vi "ex3_producer_consumer_deltat.vi"() -> ()   [LabVIEW 2022 SP3]
uses:
  C:/Program Files (x86)/National Instruments/LabVIEW 2022/examples/Connectivity/Python/support/PythonVersionsEnum.ctl
  pylabview/pythonq.lvlib
panel:
  out "delta_t_wv":dbl(graph)
  out "delta_t":dbl
  out "cur ref 2":string
  out "error out 2":errorcluster
  out "Wv 2":dbl(graph)
  out "cur ref":string
  out "count 1":i32
  in  "wait":u32=500
  out "Wv":dbl(graph)
  in  "stop":bool
  out "count 2":i32
  out "error out":errorcluster
  # "This example shows 2 connections to the python data ques, 1 to produce data, and one to consumer it, all in parrallel\n\nCreated by Jeff Morgan\nhttps://awakeniot.com/"
  # "https://github.com/jmor2000/labview_python_bridge"
  # "DATA IN"
  # "DATA OUT"
  # "DELTA T"
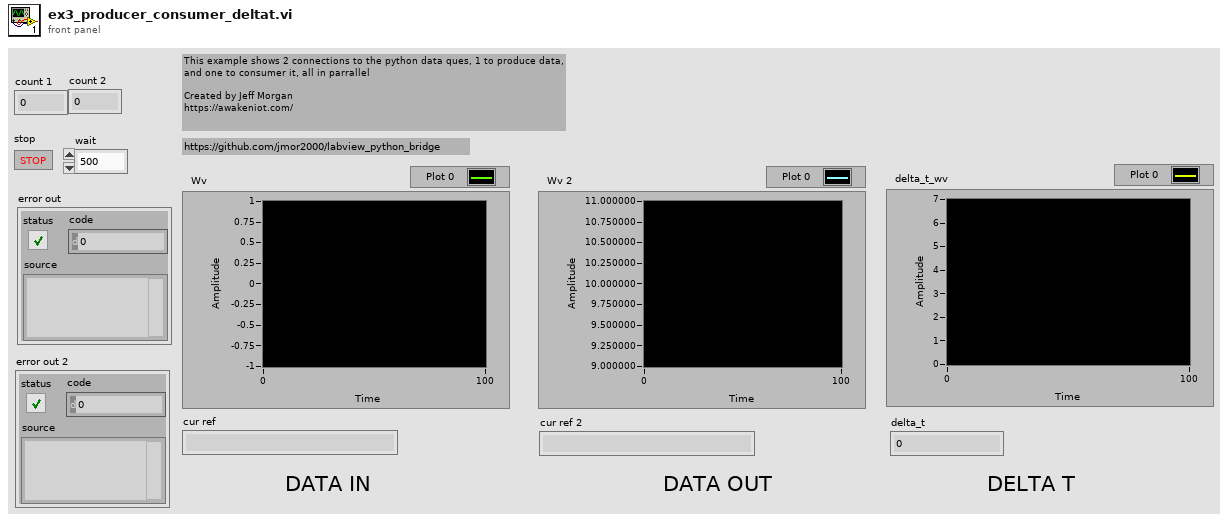
[diagram p1: front panel]
types:
  T1 = typedef "PythonVersionsEnum.ctl" = enum16{"3.6", "3.7", "3.8", "3.9"}
  T2 = typedef "pythonq.lvlib/py_cluster.ctl" = cluster{"path":path, "py":T3}
  T3 = typedef "pythonq.lvlib/py_session.ctl" = cluster{"session":refnum<k35>, "object":refnum<k38>}
  T4 = typedef "pythonq.lvlib/py_result.ctl" = cluster{"value":string, "ok":bool, "error_msg":string}
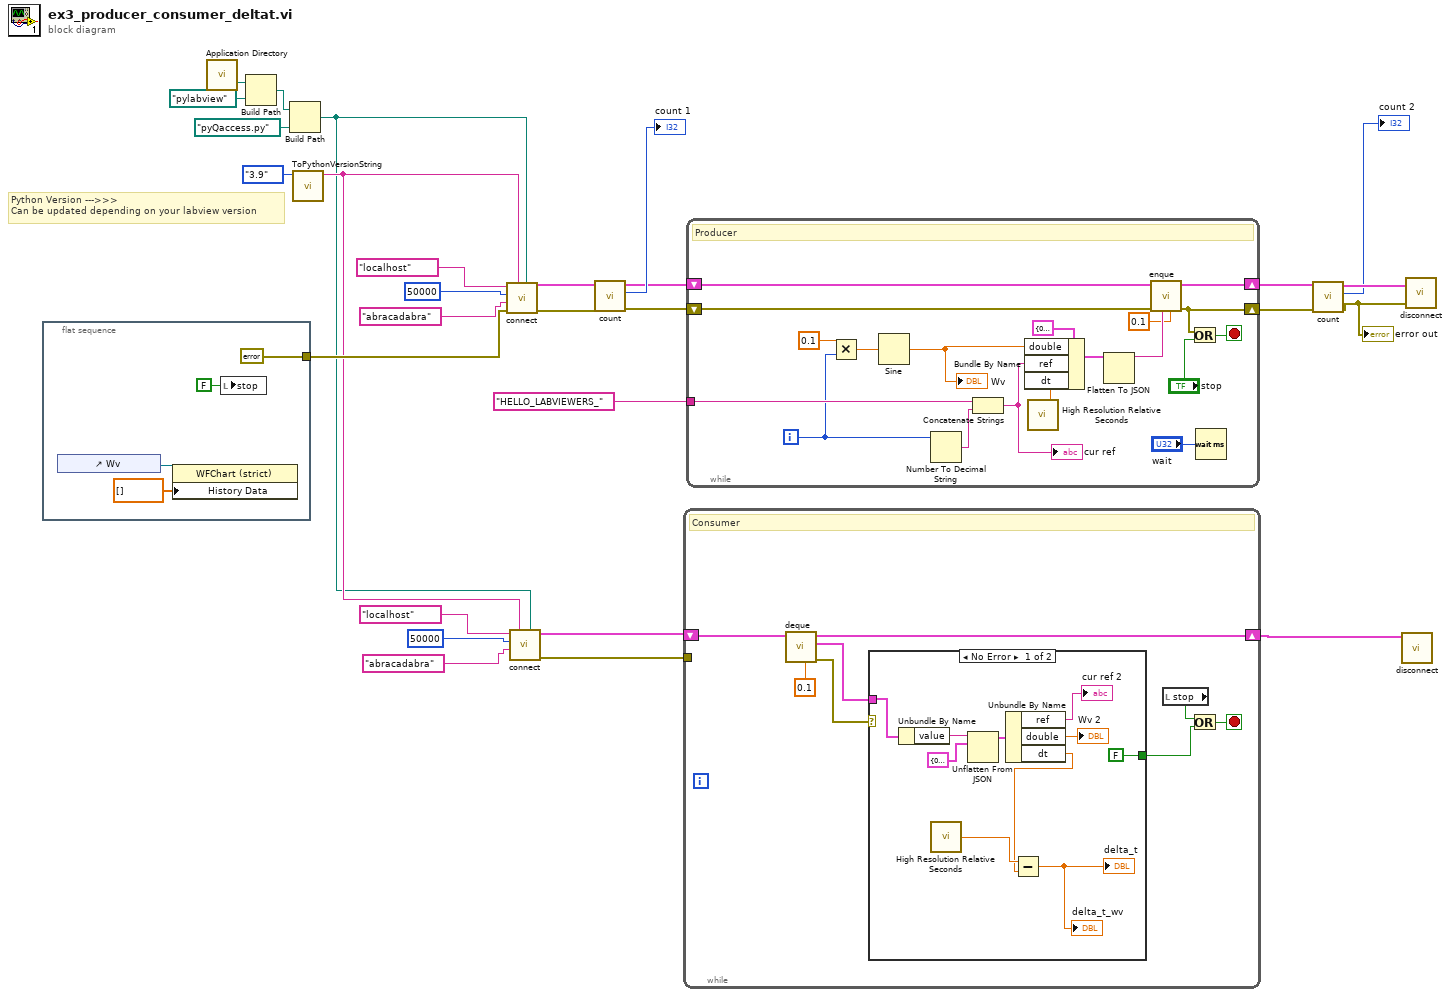
[diagram p0: block diagram]
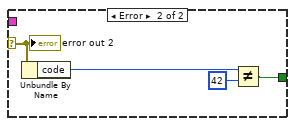
[diagram p2: hidden frame]
diagram:
  # "Python Version --->>>\nCan be updated depending on your labview version"
  n1 = flat-sequence {
    tunnel: [errorcluster {"status"=FALSE, "code"=0, "source"=""} ("error in (no error)")] -> w15
    frame #0 {
      n2 = control-ref of="Wv"() -> (w30:refnum<vi>)
      n3 = property class="WFChart (strict)"(reference=w30, "History Data"=dbl[] []) -> ()  [unwired: 1 in, 2 out]
      n4 = local write "stop"(FALSE ("stop")) -> ()
    }
  }
  n5 = call <vilib>:"Application Directory.vi"() -> ("Application Directory"=w23:path)
  n6 = Build Path(base path=w23, name or relative path=path "pylabview") -> (appended path=w24:path)
  n7 = Build Path(base path=w24, name or relative path=path "pyQaccess.py") -> (appended path=w5:path)
  n8 = call "ToPythonVersionString.vi"("python version"=PythonVersionsEnum."3.9") -> ("python version string"=w6:string)  [unwired: 10 in]
  n9 = call "connect.vi"("module path"=w5, "Python version"=w6, "error in (no error)"=w15, "password"="abracadabra", "port"=50000, "ip_address"="localhost") -> ("error out"=w18:errorcluster, "py out"=w17:T2)  [unwired: 4 in]
  n10 = call "connect.vi"("module path"=w5, "Python version"=w6, "password"="abracadabra", "port"=50000, "ip_address"="localhost") -> ("error out"=w3:errorcluster, "py out"=w4:T2)  [unwired: 5 in]
  n11 = call "count.vi"("error in (no error)"=w18, "py in"=w17) -> ("error out"=w14:errorcluster, "count"=→"count 1":i32, "py out"=w10:T2)  [unwired: 7 in]
  n12 = while {
    shift-right: [w39] -> w1
    shift-left: w4 -> [w40]
    tunnel: w3 -> [_]
    stop <- w36 stop-if-true
    # "Consumer"
    n13 = call "deque.vi"("timeout"=0.1, "py in"=w40) -> ("error out"=w37:errorcluster, "response"=w34:T4, "py out"=w39:T2)  [unwired: 6 in, 1 out]
    n14 = case shown="No Error" w37 {
      selector: w37 -> [_ w54]
      tunnel: [FALSE w51] -> w35
      tunnel: w34 -> [w49 _]
      frame No Error {
        n15 = Unbundle By Name(w49) -> ("value"=w48:string)
        n16 = call <vilib>:"High Resolution Relative Seconds.vi"() -> ("relative seconds"=w44:dbl)
        n17 = Unflatten From JSON(JSON string=w48, type and defaults=cluster{"double":dbl, "ref":string, "dt":dbl} {"double"=0.0, "ref"="", "dt"=0.0} ("Cluster")) -> (value=w47:cluster{"double":dbl, "ref":string, "dt":dbl})  [unwired: 5 in, 1 out]
        n18 = Unbundle By Name(w47) -> ("ref"=→"cur ref 2":string, "double"=→"Wv 2":dbl, "dt"=w41:dbl)
        n19 = Subtract(x=w44, y=w41) -> (x-y=→"delta_t" →"delta_t_wv":dbl)
      }
      frame Error {
        n20 = Unbundle By Name(w54) -> ("code"=w53:i32)
        n21 = Not Equal?(x=w53, y=42) -> (x != y?=w51:bool)
        "error out 2" <- w54
      }
    }
    n22 = local read "stop"() -> (w33:bool)
    n23 = Or(x=w33, y=w35) -> (x .or. y?=w36:bool)
  }
  n24 = while {
    shift-right: [w72] -> w2
    shift-left: w10 -> [w73]
    shift-right: [w69] -> w16
    shift-left: w14 -> [w71]
    tunnel: "HELLO_LABVIEWERS_" ("ref_prefix") -> [w66]
    i -> [w58]
    stop <- w70 stop-if-true
    # "Producer"
    n25 = Multiply(x=0.1, y=w58) -> (x*y=w59:dbl)
    n26 = Sine(x=w59) -> (sin(x)=w57:dbl)
    "Wv" <- w57
    n27 = Number To Decimal String(number=w58) -> (decimal integer string=w65:string)  [unwired: 1 in]
    n28 = Concatenate Strings(w66, w65) -> (w64:string)
    "cur ref" <- w64
    n29 = call <vilib>:"High Resolution Relative Seconds.vi"() -> ("relative seconds"=w55:dbl)
    n30 = Bundle By Name(cluster=cluster{"double":dbl, "ref":string, "dt":dbl} {"double"=0.0, "ref"="", "dt"=0.0} ("Cluster"), "double"=w57, "ref"=w64, "dt"=w55) -> (w63:cluster{"double":dbl, "ref":string, "dt":dbl})
    n31 = Flatten To JSON(anything=w63) -> (JSON string=w62:string)  [unwired: 2 in, 1 out]
    n32 = call "enque.vi"("timeout"=0.1, "data in"=w62, "error in (no error)"=w71, "py in"=w73) -> ("error out"=w69:errorcluster, "py out"=w72:T2)  [unwired: 4 in, 2 out]
    n33 = Or(x=w69, y="stop") -> (x .or. y?=w70:bool)
    n34 = Wait (ms)(milliseconds to wait="wait") -> ()  [unwired: 1 out]
  }
  n35 = call "count.vi"("error in (no error)"=w16, "py in"=w2) -> ("error out"=w12:errorcluster, "count"=→"count 2":i32, "py out"=w20:T2)  [unwired: 7 in]
  "error out" <- w12
  n36 = call "disconnect.vi"("py in"=w1) -> ()  [unwired: 10 in, 1 out]
  n37 = call "disconnect.vi"("error in (no error)"=w12, "py in"=w20) -> ()  [unwired: 9 in, 1 out]
